vi "re_sig.stop_lua.vi"(5 "LuaVIEW reference":T1) -> (15 "error out":errorcluster)   [LabVIEW 2012]
doc: "Sets the \"stop\" signal of the specified task if allowed by that task. To reduce response latency, the task being signalled is woken up when asleep. Note that this call is asynchronous: the signal might not have been handled yet when this call returns.\nParameters:\nstr:task_identifier"
uses:
  typedefs/t_LuaVIEW Reference.ctl
  typedefs/t_LuaVIEW Task List Methods.ctl
  subvis/private/LuaVIEW Pull (string).vi
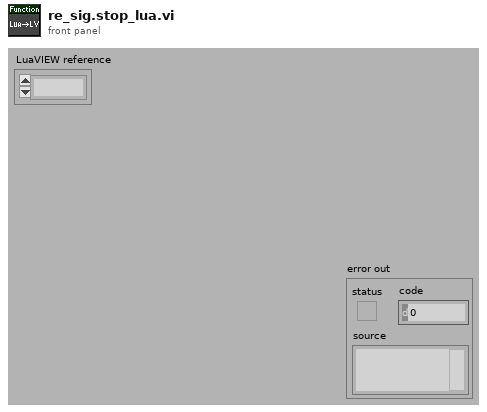
[diagram p1: front panel]
types:
  T1 = typedef "t_LuaVIEW Reference.ctl" = refnum<k1>
  T2 = typedef "t_LuaVIEW Task List Methods.ctl" = enum16{"clear list", "add", "test", "remove", "get ref", "get task info", "get list", "get script info", "ongoing?", "resume", "pause", "stop", "confirm", "message"}
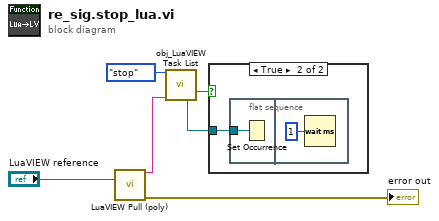
[diagram p0: block diagram]
diagram:
  n1 = call-poly "LuaVIEW Pull (poly).vi"("LuaVIEW reference in"="LuaVIEW reference") -> ("string"=w3:string, "error out"=→"error out":errorcluster)  [unwired: 12 in, 1 out]
  n2 = call "obj_LuaVIEW Task List.vi"("method"=t_LuaVIEW_Task_List_Methods."stop", "task identifier"=w3) -> ("set/ongoing"=w5:bool, "wakeup occurrence"=w4:refnum<k4>)  [unwired: 8 in, 4 out]
  n3 = case shown="True" w5 {
    tunnel: w4 -> [_ w7]
    frame False {
    }
    frame True {
      n4 = flat-sequence {
        tunnel: w7 -> [w8]
        frame #0 {
          n5 = Set Occurrence(w8) -> ()
        }
        frame #1 {
          n6 = Wait (ms)(milliseconds to wait=u32 1) -> ()  [unwired: 1 out]
        }
      }
    }
  }
